vi "TDCTime.vi"(1 "Enum":enum16{"Get", "Init"}(ring)) -> (0 "TDCTime":i32)   [LabVIEW 2016]
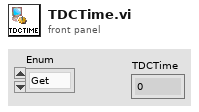
[diagram p1: front panel]
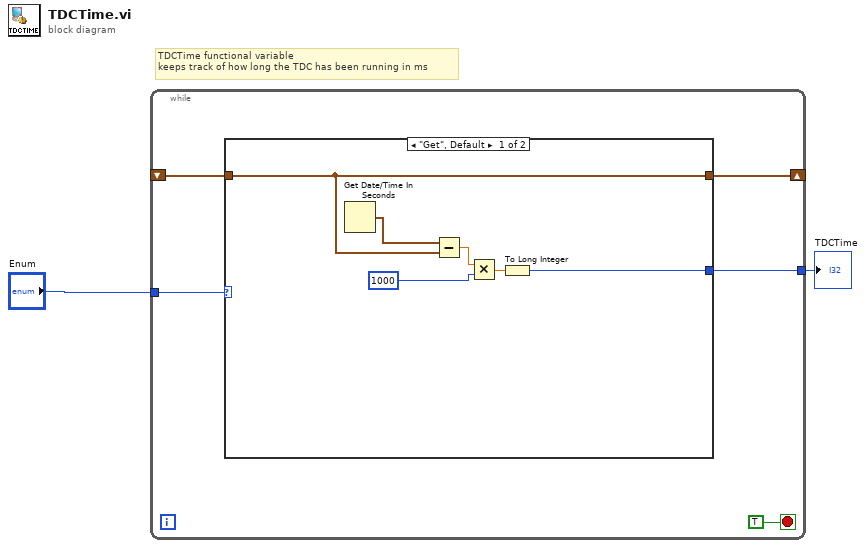
[diagram p0: block diagram]
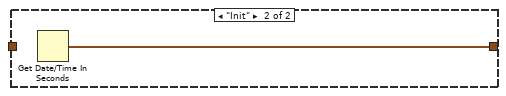
[diagram p2: hidden frame]
diagram:
  # "TDCTime functional variable\nkeeps track of how long the TDC has been running in ms"
  n1 = while {
    tunnel: "Enum" -> [w7]
    shift-right: [w6] -> _
    shift-left: _ -> [w5]
    tunnel: [w4] -> w1
    stop <- TRUE stop-if-true
    n2 = case shown="\"Get\", Default" w7 {
      tunnel: [w13 w14] -> w6
      tunnel: w5 -> [w13 _]
      tunnel: [w9 _] -> w4
      frame "Get", Default {
        n3 = Get Date/Time In Seconds() -> (seconds since 1Jan1904=w8:timestamp)
        n4 = Subtract(x=w8, y=w13) -> (x-y=w12:dbl)
        n5 = Multiply(x=w12, y=i64 1000) -> (x*y=w10:dbl)
        n6 = To Long Integer(number=w10) -> (32bit integer=w9:i32)
      }
      frame "Init" {
        n7 = Get Date/Time In Seconds() -> (seconds since 1Jan1904=w14:timestamp)
      }
    }
  }
  "TDCTime" <- w1
